vi "String EW.vi"(11 "Data In":string) -> (3 "Data Out":string)   [LabVIEW 2018]
uses:
  Core/Assert API Components/Failure Actions.ctl
  Core/Assert API Components/Assert API Components.lvlib
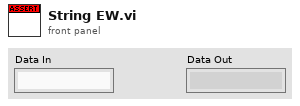
[diagram p1: front panel]
types:
  T1 = typedef "Assert API Components.lvlib/Failure Actions.ctl" = enum16{"None", "Log To File", "Pause Execution", "Abort Execution"}
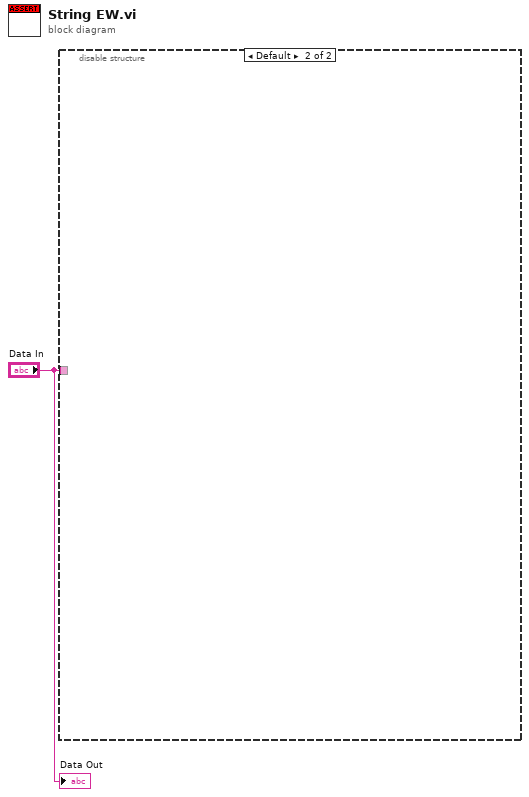
[diagram p0: block diagram]
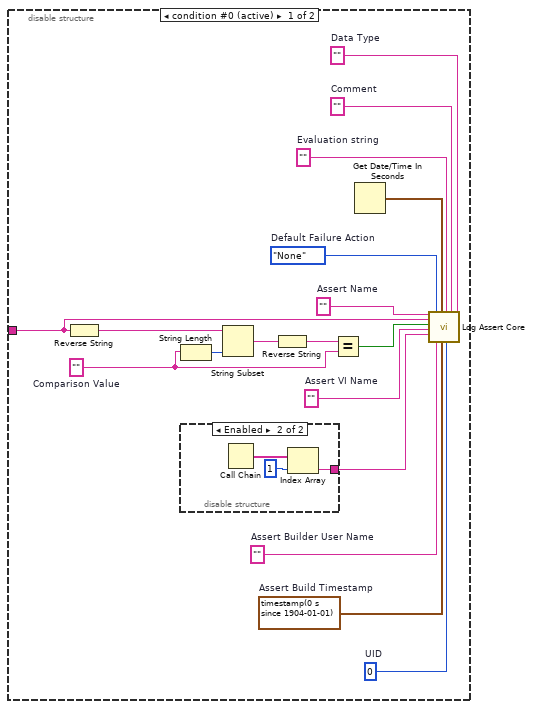
[diagram p2: hidden frame]
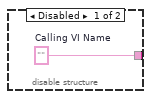
[diagram p3: hidden frame]
diagram:
  n1 = disable-structure shown="Default" {
    disable-tunnel: "Data In" -> [w15 _]
    frame condition #0 (active) {
      w3 = 0  # UID
      w5 = ""  # Assert VI Name
      w6 = ""  # Data Type
      w7 = ""  # Assert Builder User Name
      w8 = timestamp(0 s since 1904-01-01)  # Assert Build Timestamp
      w17 = ""  # Comment
      w16 = ""  # Evaluation string
      w18 = Failure_Actions."None"  # Default Failure Action
      w19 = ""  # Assert Name
      w12 = ""  # Comparison Value
      n2 = Reverse String(1:w15) -> (0:w10:string)
      n3 = String Length(string=w12) -> (length=w14:i32)
      n4 = disable-structure shown="Enabled" {
        disable-tunnel: [w20 w21] -> w2
        frame Disabled {
          w20 = ""  # Calling VI Name
        }
        frame Enabled {
          n5 = Call Chain() -> (call chain=w22:string[])
          n6 = Index Array(array=w22, index=1) -> (element=w21:string)
        }
      }
      n7 = String Subset(string=w10, length (rest)=w14) -> (substring=w13:string)  [unwired: 1 in]
      n8 = Reverse String(1:w13) -> (0:w9:string)
      n9 = Equal?(x=w9, y=w12) -> (x = y?=w11:bool)
      n10 = Get Date/Time In Seconds() -> (seconds since 1Jan1904=w4:timestamp)
      n11 = call "Log Assert Core.vi"("Assert Name"=w19, "Data Value"=w15, "Status"=w11, "Assert VI Name"=w5, "Calling VI Name"=w2, "Failure Action"=w18, "Assert Builder User Name"=w7, "Last Update"=w4, "Assert Build Timestamp"=w8, "Evaluation String"=w16, "Assert VI UID"=w3, "Comment"=w17, "Data Type"=w6) -> ()  [unwired: 7 in]
    }
    frame condition #1 {
    }
  }
  "Data Out" <- "Data In"
